vi "Climb_Pivot_Execute.vi"   [LabVIEW 2019]
uses:
  Globals/Climb_Globals.vi
  <vilib>/Rock Robotics/WPI/ThirdParty/REV Robotics/SPARK MAX/Typedef/Spark MAX Control Type.ctl
types:
  T1 = typedef "WPI_MotorControlDeviceRef.ctl" = cluster{"DeviceStatus":errorcluster, "Type":T2, "PWM":cluster{"PWM Channel":T3, "DeadBand":T4}, "CAN":cluster{"Device Number":u8, "SetOutput VI Ref":variant, "GetOutput VI Ref":variant, "Enable VI Ref":variant, "Disable VI Ref":variant, "Data":variant}, "Invert":bool, "DIO PWM":cluster{"PWM \"Enable\" Channel":T3, "DIOChannel":T5, "PWM Rate":dbl}}
  T2 = typedef "WPI_MotorControlType.ctl" = enum16{"PWM", "CAN", "DIO PWM"}
  T3 = typedef "FPGA_DIOPWMChannel.ctl" = enum8{"PWM 0", "PWM 1", "PWM 2", "PWM 3", "PWM 4", "PWM 5", "PWM 6", "PWM 7", "PWM 8", "PWM 9", "PWM MXP 0", "PWM MXP 1", "PWM MXP 2", "PWM MXP 3", "PWM MXP 4", "PWM MXP 5", "PWM MXP 6", "PWM MXP 7", "PWM MXP 8", "PWM MXP 9", "Invalid"}
  T4 = typedef "WPI_PWMDeadband.ctl" = cluster{"Name":string, "maxPositivePwm":i32, "minPositivePwm":i32, "centerPwm":i32, "maxNegativePwm":i32, "minNegativePwm":i32, "angularRange":u16}
  T5 = typedef "FPGA_DIOChannel.ctl" = enum8{"DIO 0", "DIO 1", "DIO 2", "DIO 3", "DIO 4", "DIO 5", "DIO 6", "DIO 7", "DIO 8", "DIO 9", "DIO MXP 0", "DIO MXP 1", "DIO MXP 2", "DIO MXP 3", "DIO MXP 4", "DIO MXP 5", "DIO MXP 6", "DIO MXP 7", "DIO MXP 8", "DIO MXP 9", "DIO MXP 10", "DIO MXP 11", "DIO MXP 12", "DIO MXP 13", "DIO MXP 14", "DIO MXP 15", "SPI Port CS1", "SPI Port CS2", "SPI Port CS3", "SPI Port MISO", "SPI Port MOSI", "Invalid"}
  T6 = typedef "Spark MAX Control Type.ctl" = enum16{"Percent VBus", "Voltage", "Velocity", "Position", "Smart Motion", "Current", "Smart Velocity"}
  T7 = typedef "Climb_Pivot_Cluster.ctl" = cluster{"Up?":bool, "Pivot_Throttle":dbl, "Control_States":T8}
  T8 = typedef "Climb_Pivot_Control_States.ctl" = enum16{"No-Op", "Moving_Down", "Moving_Up", "Manual"}
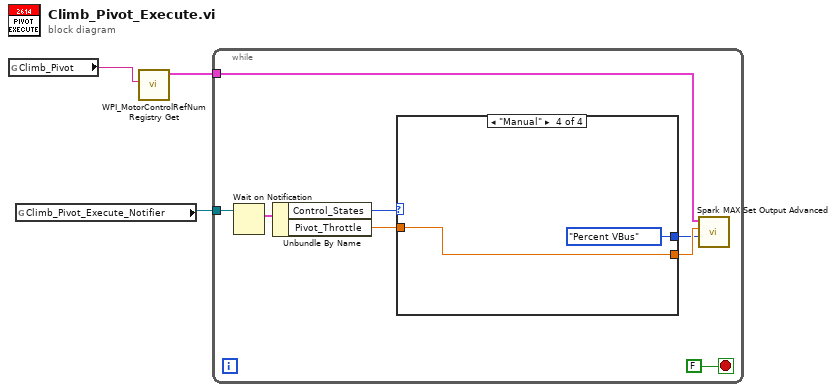
[diagram p0: block diagram]
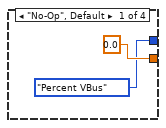
[diagram p2: hidden frame]
diagram:
  n1 = global read "Climb_Globals.vi" "Climb_Pivot"() -> (w2:string)
  n2 = global read "Climb_Globals.vi" "Climb_Pivot_Execute_Notifier"() -> (w3:refnum<notifier>)
  n3 = call <vilib>:"WPI_MotorControlRefNum Registry Get.vi"("refnum name"=w2) -> ("MotorControlDevRef"=w1:T1)  [unwired: 9 in, 1 out]
  n4 = while {
    tunnel: w3 -> [w10]
    tunnel: w1 -> [w7]
    stop <- FALSE stop-if-true
    n5 = Wait on Notification(notifier=w10) -> (notification=w9:T7)  [unwired: 3 in, 3 out]
    n6 = Unbundle By Name(w9) -> ("Control_States"=w8:T8, "Pivot_Throttle"=w4:dbl)
    n7 = case shown="\"Manual\"" w8 {
      tunnel: [0.0 ("Arbitrary Feed Forward (0)") _ _ w14] -> w6
      tunnel: [Spark_MAX_Control_Type."Percent VBus" ("Control Mode") _ _ Spark_MAX_Control_Type."Percent VBus" ("Control Mode")] -> w5
      tunnel: w4 -> [_ _ _ w14]
      frame "No-Op", Default {
      }
      frame "Moving_Down" {
      }
      frame "Moving_Up" {
      }
      frame "Manual" {
      }
    }
    n8 = call <vilib>:"Spark MAX Set Output Advanced.vi"("Control Mode"=w5, "Setpoint"=w6, "MotorControlDevRef"=w7) -> ()  [unwired: 7 in, 2 out]
  }
